vi "create TCP connection.vi"(8 "error in":errorcluster, 10 "connection":refnum<k5>) -> (0 "error out":errorcluster, 3 "TCP connection out":refnum<class "TCP connection.lvclass">)   [LabVIEW 2015, in "TCP connection.lvclass"]
uses:
  TCP connection.lvclass
  TCP connection.lvclass/TCP connection.ctl
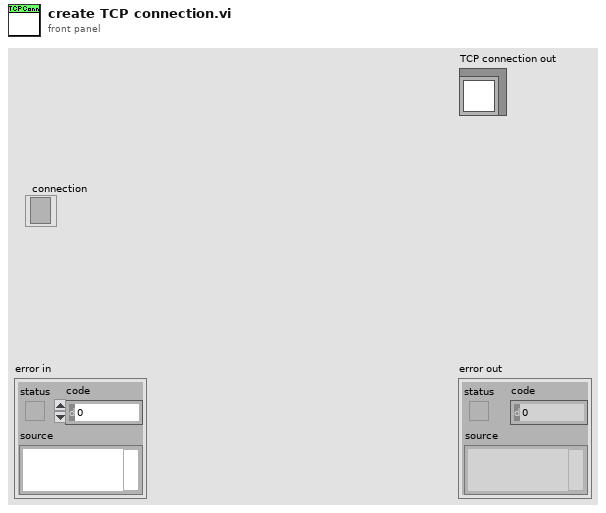
[diagram p1: front panel]
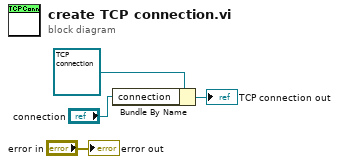
[diagram p0: block diagram]
diagram:
  n1 = Bundle By Name(cluster=refnum<class "TCP connection.lvclass"> refnum ("TCP connection in"), "connection"="connection") -> (→"TCP connection out":refnum<class "TCP connection.lvclass">)
  "error out" <- "error in"
